vi "Array2Fifo.vi"(9 "Input Array":dbl[](array[numeric]), 11 "rt fifo":refnum<k33>) -> ()   [LabVIEW 2010, in "KevLib01.lvlib"]
uses:
  KevLib01.lvlib
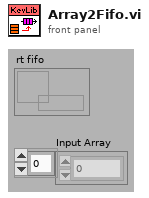
[diagram p1: front panel]
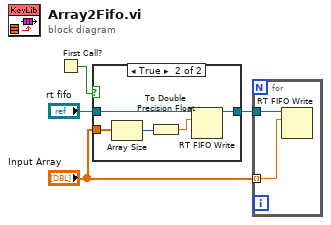
[diagram p0: block diagram]
diagram:
  n1 = First Call?() -> (First Call?: T/F=w4:bool)
  n2 = case shown="True" w4 {
    tunnel: "rt fifo" -> [w5 w10]
    tunnel: [w5 w9] -> w1
    tunnel: "Input Array" -> [_ w8]
    frame False {
    }
    frame True {
      n3 = Array Size(array=w8) -> (size(s)=w6:i32)
      n4 = To Double Precision Float(number=w6) -> (double precision float=w7:dbl)
      n5 = RT FIFO Write(0:w10, 1:w7) -> (8:w9:refnum<k33>)  [unwired: 2 in, 4 out]
    }
  }
  n6 = for {
    tunnel: "Input Array" -> [w11] mode=indexing
    tunnel: w1 -> [w12]
    n7 = RT FIFO Write(0:w12, 1:w11) -> ()  [unwired: 2 in, 5 out]
  }
